vi "2012_01_17 Flow Crunch.vi"(6 "Capture":bool, 7 "Motor #":i32, 8 "error in (no error)":errorcluster, 9 "data":waveform(dbl)[](array[waveform]), 10 "Elapsed Time (s)":dbl, 11 "Motor In":T1={"Fail"=FALSE, "RPM"=0, "Motor"=enum."Maxon EC6 6V", "ESC"=enum."Phoenix 10", "Supply (V)"=0.0, "Elapsed Time"=0.0, "Counter"=0.0, "Torque (mNm)"=0.0, "Electrical Power (W)"=0.0, "Motor Efficiency"=0.0, "Mechanical Power (W)"=0.0, "Supply Power (W)"=0.0, "ESC Efficiency"=0.0, "PWM"=0, "Direction"=enum."Push"} {"PWM" min=0 max=100 step=1 scale=0.0..100.0; "ESC Efficiency" format="%#_3g%%"; "Supply Power (W)" format="%.3g"; "Mechanical Power (W)" format="%.3g"; "Motor Efficiency" format="%#_3g%%"; "Electrical Power (W)" format="%.3g"; "Torque (mNm)" format="%.3g"; "Elapsed Time" format="%<%H:%M:%S>t"; "Supply (V)" format="%.2f"; "RPM" scale=0.0..60000.0}) -> (0 "error out":errorcluster, 2 "Dynamic Data Type":dynamicdata(waveform), 3 "Motor Out":T1={"Fail"=FALSE, "RPM"=0, "Motor"=enum."Maxon EC6 6V", "ESC"=enum."Phoenix 10", "Supply (V)"=0.0, "Elapsed Time"=0.0, "Counter"=0.0, "Torque (mNm)"=0.0, "Electrical Power (W)"=0.0, "Motor Efficiency"=0.0, "Mechanical Power (W)"=0.0, "Supply Power (W)"=0.0, "ESC Efficiency"=0.0, "PWM"=0, "Direction"=enum."Push"} {"PWM" min=0 max=100 step=1 scale=0.0..100.0; "ESC Efficiency" format="%#_3g%%"; "Supply Power (W)" format="%.3g"; "Mechanical Power (W)" format="%.3g"; "Motor Efficiency" format="%#_3g%%"; "Electrical Power (W)" format="%.3g"; "Torque (mNm)" format="%.3g"; "Elapsed Time" format="%<%H:%M:%S>t"; "Supply (V)" format="%.2f"; "RPM" scale=0.0..60000.0})   [LabVIEW 2013]
uses:
  Flow Type Def.ctl
  <vilib>/measure/madcrms.llb/Basic Averaged DC-RMS for 1 Chan.vi
  <vilib>/measure/matone.llb/Extract Single Tone Information 1 Chan.vi
  <vilib>/express/express arith-compare/Formula/XNode/ExpressFormulaBlockNode.xnode
  <vilib>/measure/NI_MAPro.lvlib
panel:
  # "Stopped"
  # "Stopped"
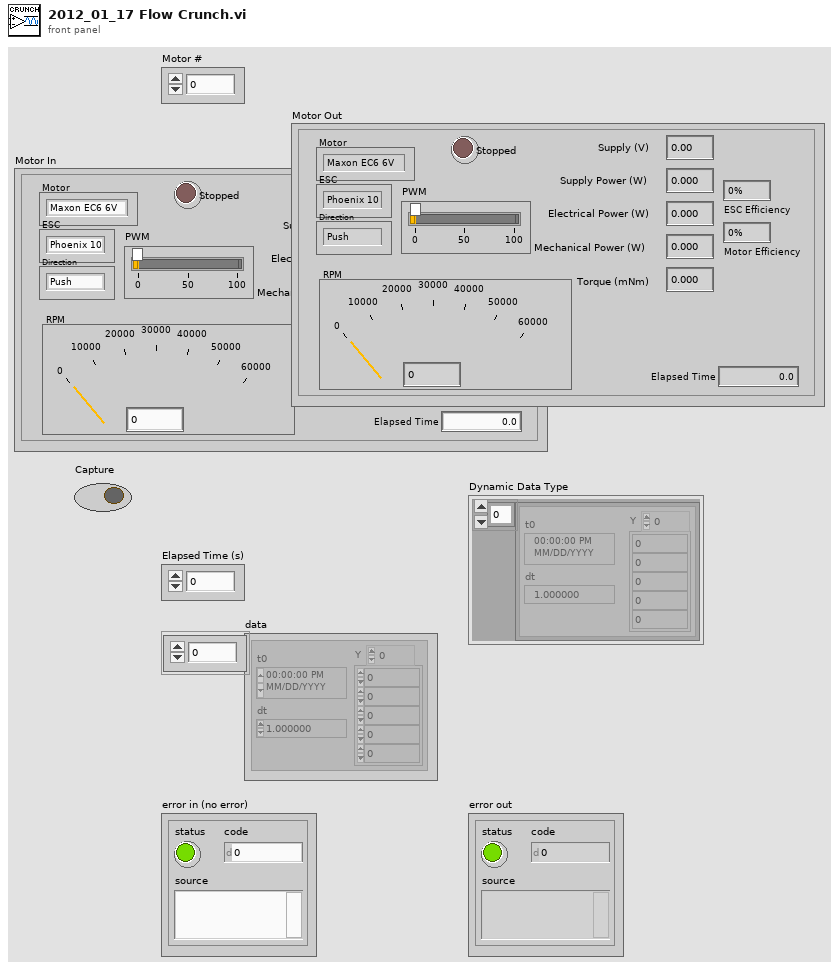
[diagram p1: front panel]
types:
  T1 = typedef "Flow Type Def.ctl" = cluster{"Fail":bool, "RPM":u64, "Motor":enum16{"", "Maxon EC6 6V", "Maxon EC4 6V", "FH 0620 6V", "FH 0620 12V", "FH 0427"}, "ESC":enum16{"Phoenix 10", "Maxon", "FH 1801"}, "Supply (V)":dbl, "Elapsed Time":dbl, "Counter":dbl, "Torque (mNm)":dbl, "Electrical Power (W)":dbl, "Motor Efficiency":dbl, "Mechanical Power (W)":dbl, "Supply Power (W)":dbl, "ESC Efficiency":dbl, "PWM":i32, "Direction":enum16{"Push", "Pull"}}
  T2 = enum16{"", "Maxon EC6 6V", "Maxon EC4 6V", "FH 0620 6V", "FH 0620 12V", "FH 0427"}
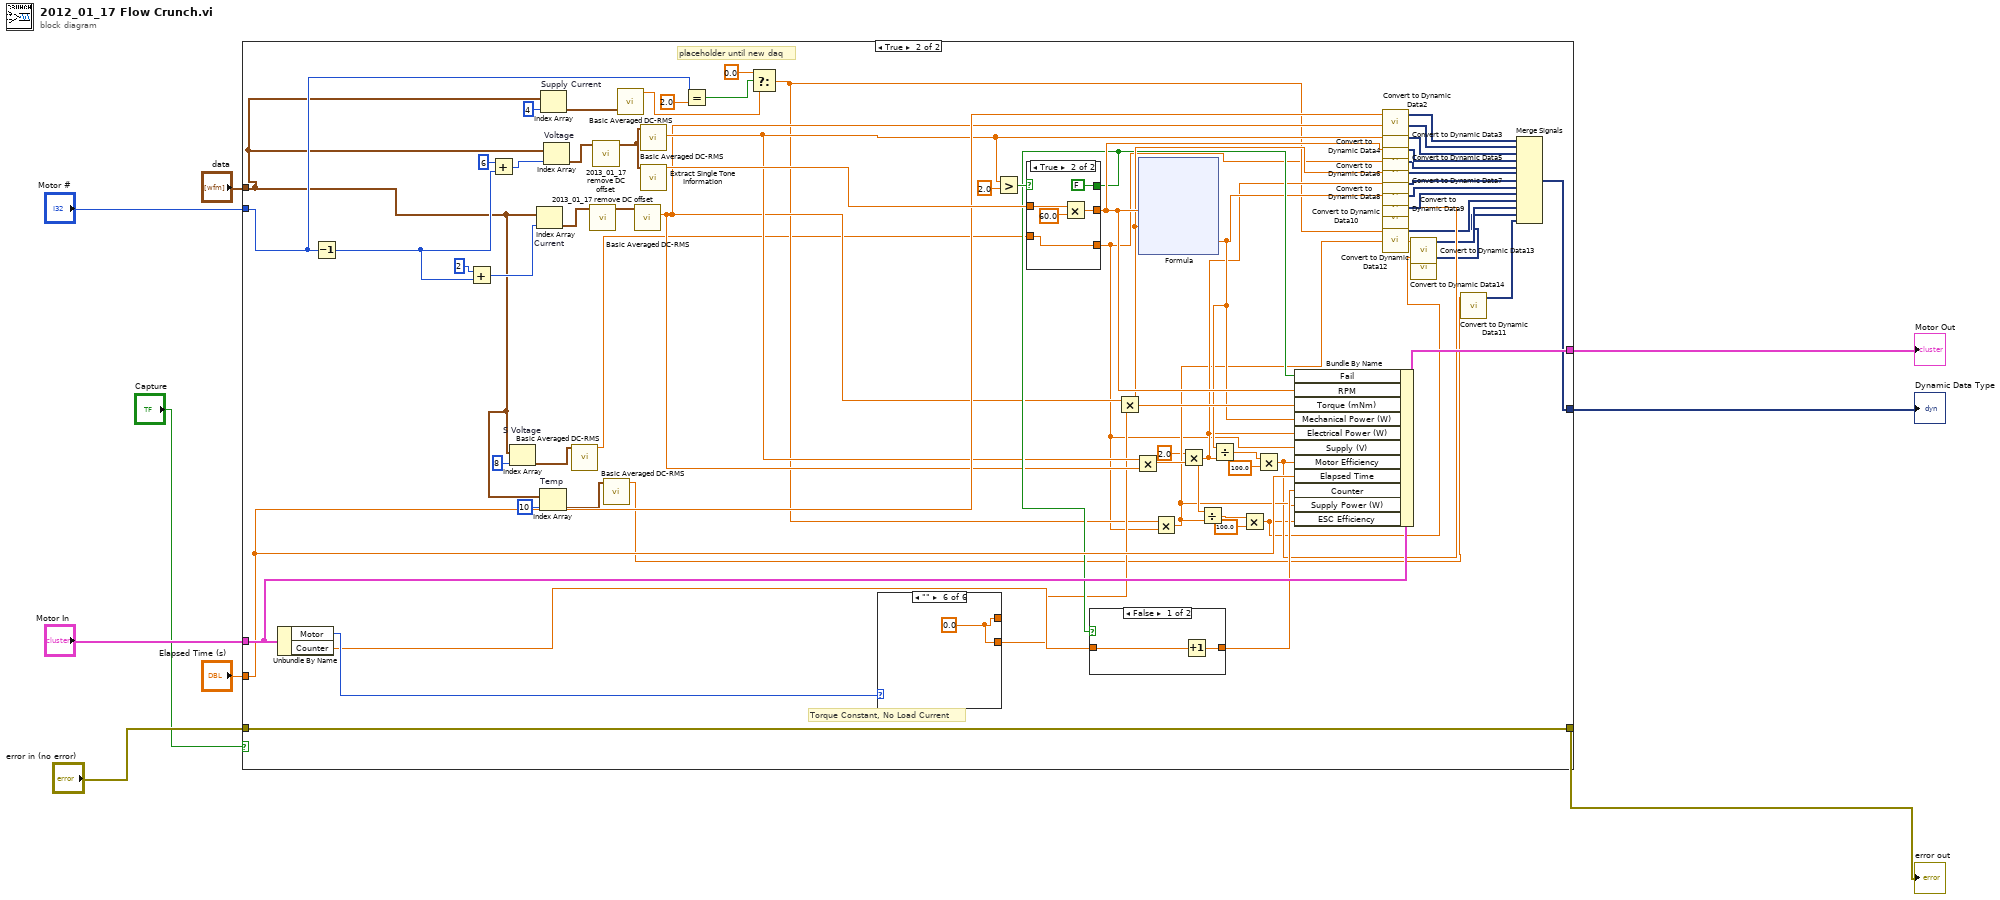
[diagram p0: block diagram]
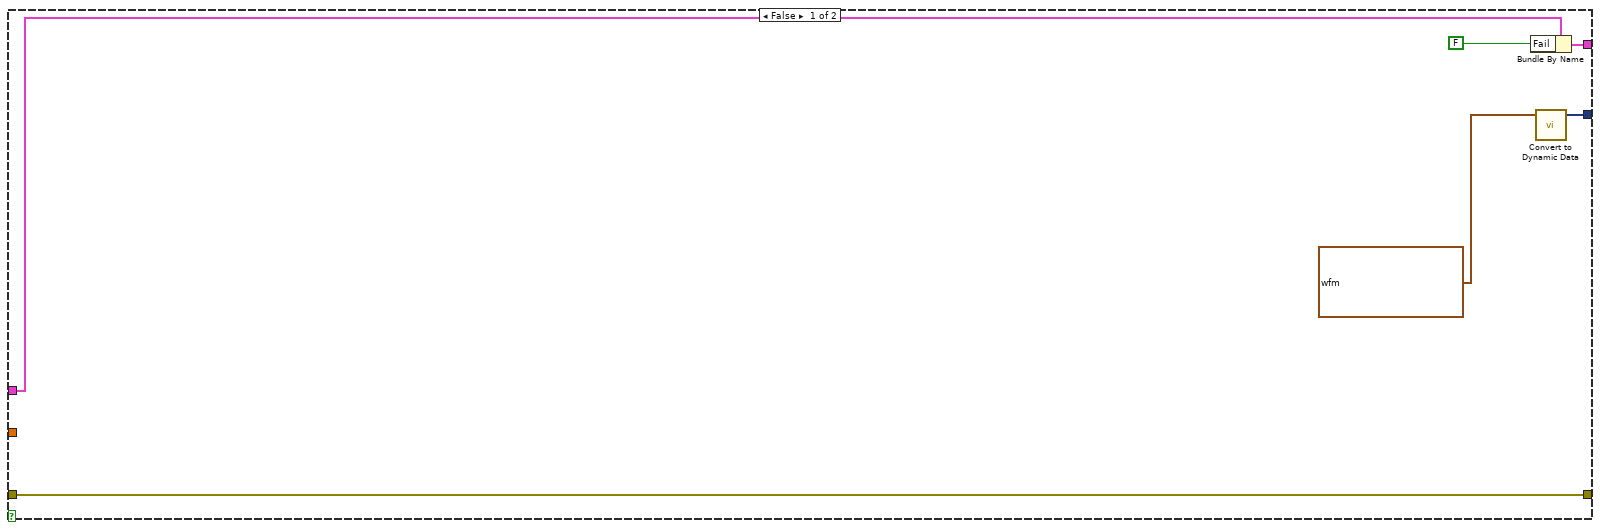
[diagram p2: hidden frame]
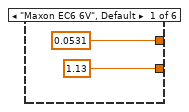
[diagram p4: hidden frame]
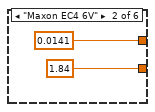
[diagram p5: hidden frame]
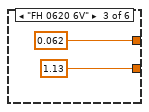
[diagram p6: hidden frame]
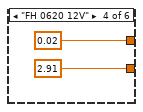
[diagram p7: hidden frame]
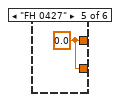
[diagram p8: hidden frame]
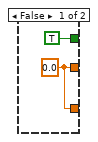
[diagram p9: hidden frame]
diagram:
  n1 = case shown="True" "Capture" {
    tunnel: "Motor #" -> [_ w40]
    tunnel: "Motor In" -> [w15 w77]
    tunnel: [w14 w76] -> w3
    tunnel: "data" -> [_ w20]
    tunnel: "error in (no error)" -> [w12 w75]
    tunnel: [w12 w75] -> w6
    tunnel: "Elapsed Time (s)" -> [_ w71]
    tunnel: [w10 w60] -> w8
    frame False {
      n2 = Bundle By Name(cluster=w15, "Fail"=FALSE) -> (w14:T1)
      n3 = call "Convert to Dynamic Data"("Waveform"=waveform(dbl) {"t0"=timestamp(0 s since 1904-01-01), "dt"=1.0, "Y"=[]}) -> ("Dynamic Data Type"=w10:dynamicdata)  [unwired: 3 in]
    }
    frame True {
      # "placeholder until new daq"
      # "Torque Constant, No Load Current"
      n4 = Unbundle By Name(w77) -> ("Motor"=w78:T2, "Counter"=w74:dbl)
      n5 = Decrement(x=w40) -> (x-1=w31:i32)
      n6 = Add(x=2 ("index"), y=w31) -> (x+y=w30:i32)
      n7 = Add(x=6 ("index"), y=w31) -> (x+y=w33:i32)
      n8 = Index Array "S Voltage"(array=w20, index=8) -> (element=w22:waveform(dbl))
      n9 = Index Array "Current"(array=w20, index=w30) -> (element=w58:waveform(dbl))
      n10 = Index Array "Temp"(array=w20, index=10) -> (element=w18:waveform(dbl))
      n11 = Index Array "Supply Current"(array=w20, index=4) -> (element=w54:waveform(dbl))
      n12 = Index Array "Voltage"(array=w20, index=w33) -> (element=w56:waveform(dbl))
      n13 = call-poly <vilib>:"Basic Averaged DC-RMS.vi"("signal in"=w22) -> ("DC value"=w21:dbl)  [unwired: 7 in, 3 out]
      n14 = call "2013_01_17 remove DC offset.vi"("Waveform in"=w58) -> ("Waveform out"=w57:waveform(dbl))  [unwired: 10 in]
      n15 = call "2013_01_17 remove DC offset.vi"("Waveform in"=w56) -> ("Waveform out"=w28:waveform(dbl))  [unwired: 10 in]
      n16 = call-poly <vilib>:"Basic Averaged DC-RMS.vi"("signal in"=w18) -> ("DC value"=w17:dbl)  [unwired: 7 in, 3 out]
      n17 = call-poly <vilib>:"Basic Averaged DC-RMS.vi"("signal in"=w54) -> ("DC value"=w37:dbl)  [unwired: 7 in, 3 out]
      n18 = call-poly <vilib>:"Basic Averaged DC-RMS.vi"("signal in"=w57) -> ("RMS value"=w43:dbl)  [unwired: 7 in, 3 out]
      n19 = call-poly <vilib>:"Basic Averaged DC-RMS.vi"("signal in"=w28) -> ("RMS value"=w44:dbl)  [unwired: 7 in, 3 out]
      n20 = call-poly <vilib>:"Extract Single Tone Information.vi"("time signal in"=w28) -> ("detected frequency"=w79:dbl)  [unwired: 5 in, 5 out]
      n21 = Equal?(x=w40, y=2.0) -> (x = y?=w39:bool)
      n22 = Select(t=0.0, s=w39, f=w37) -> (s? t:f=w36:dbl)
      n23 = case shown="\"\"" w78 {
        tunnel: [1.13 1.84 1.13 2.91 w103 w104] -> w42
        tunnel: [0.0531 0.0141 0.062 0.02 w103 w104] -> _
        frame "Maxon EC6 6V", Default {
        }
        frame "Maxon EC4 6V" {
        }
        frame "FH 0620 6V" {
        }
        frame "FH 0620 12V" {
        }
        frame "FH 0427" {
          w103 = 0.0
        }
        frame "" {
          w104 = 0.0
        }
      }
      n24 = Greater?(x=w44, y=2.0) -> (0:w81:bool)
      n25 = case shown="True" w81 {
        tunnel: [w105 w111] -> w73
        tunnel: w79 -> [_ w109]
        tunnel: [TRUE FALSE] -> w59
        tunnel: [w105 w107] -> w27
        tunnel: w21 -> [_ w107]
        frame False {
          w105 = 0.0 ("y")
        }
        frame True {
          n26 = Multiply(x=w109, y=60.0) -> (x*y=w111:dbl)
        }
      }
      n27 = case shown="False" w59 {
        tunnel: w74 -> [w83 w84]
        tunnel: [w82 w84] -> w70
        frame False {
          n28 = Increment(x=w83) -> (x+1=w82:dbl)
        }
        frame True {
        }
      }
      n29 = Multiply(x=w43, y=w42) -> (x*y=w72:dbl)
      n30 = Multiply(x=w44, y=w43) -> (x*y=w55:dbl)
      n31 = xnode "Formula"("RPM"=w73, "Torque"=w72) -> ("Result"=w53:dbl)  [unwired: 1 in, 1 out]
      n32 = Multiply(x=w36, y=w27) -> (x*y=w51:dbl)
      n33 = Multiply(x=2.0, y=w55) -> (x*y=w52:dbl)
      n34 = Divide(x=w52, y=w51) -> (x/y=w46:dbl)
      n35 = Divide(x=w53, y=w52) -> (x/y=w48:dbl)
      n36 = Multiply(x=w46, y=100.0) -> (x*y=w45:dbl)
      n37 = Multiply(x=w48, y=100.0) -> (x*y=w47:dbl)
      n38 = Bundle By Name(cluster=w77, "Fail"=w59, "RPM"=w73, "Torque (mNm)"=w72, "Mechanical Power (W)"=w53, "Electrical Power (W)"=w52, "Supply (V)"=w27, "Motor Efficiency"=w47, "Elapsed Time"=w71, "Counter"=w70, "Supply Power (W)"=w51, "ESC Efficiency"=w45) -> (w76:T1)
      n39 = call "Convert to Dynamic Data2"("Double"=w71) -> ("Dynamic Data Type"=w69:dynamicdata)  [unwired: 3 in]
      n40 = call "Convert to Dynamic Data3"("Double"=w43) -> ("Dynamic Data Type"=w68:dynamicdata)  [unwired: 3 in]
      n41 = call "Convert to Dynamic Data4"("Double"=w44) -> ("Dynamic Data Type"=w67:dynamicdata)  [unwired: 3 in]
      n42 = call "Convert to Dynamic Data5"("Double"=w73) -> ("Dynamic Data Type"=w66:dynamicdata)  [unwired: 3 in]
      n43 = call "Convert to Dynamic Data6"("Double"=w27) -> ("Dynamic Data Type"=w65:dynamicdata)  [unwired: 3 in]
      n44 = call "Convert to Dynamic Data7"("Double"=w72) -> ("Dynamic Data Type"=w64:dynamicdata)  [unwired: 3 in]
      n45 = call "Convert to Dynamic Data8"("Double"=w52) -> ("Dynamic Data Type"=w63:dynamicdata)  [unwired: 3 in]
      n46 = call "Convert to Dynamic Data9"("Double"=w53) -> ("Dynamic Data Type"=w62:dynamicdata)  [unwired: 3 in]
      n47 = call "Convert to Dynamic Data10"("Double"=w47) -> ("Dynamic Data Type"=w61:dynamicdata)  [unwired: 3 in]
      n48 = call "Convert to Dynamic Data12"("Double"=w36) -> ("Dynamic Data Type"=w26:dynamicdata)  [unwired: 3 in]
      n49 = call "Convert to Dynamic Data13"("Double"=w51) -> ("Dynamic Data Type"=w25:dynamicdata)  [unwired: 3 in]
      n50 = call "Convert to Dynamic Data14"("Double"=w45) -> ("Dynamic Data Type"=w24:dynamicdata)  [unwired: 3 in]
      n51 = call "Convert to Dynamic Data11"("Double"=w17) -> ("Dynamic Data Type"=w16:dynamicdata)  [unwired: 3 in]
      n52 = Merge Signals(w69, w68, w67, w66, w65, w64, w63, w62, w61, w26, w25, w24, w16) -> (w60:dynamicdata)
    }
  }
  "Dynamic Data Type" <- w8
  "error out" <- w6
  "Motor Out" <- w3
